vi "Car Simulation.vi"() -> ()   [LabVIEW 2020]
uses:
  <vilib>/event_ctls.llb/eventvkey.ctl
  <vilib>/numeric/Random Number (Range) I64.vi
  <vilib>/numeric/sub_Random U32.vi
panel:
  out "realdir":dbl format="%#_3g"
  in  "no road/road?":bool=TRUE
  out "velocity":cluster{"x":dbl, "y":dbl}
  in  "VKey 2":T1=enum."Ctrl"
  in  "Backward?":bool
  out "String":string
  out "location":T2
  out "readings":T3
  out "buffer":T4
  in  "y buffer":dbl
  in  "x buffer":dbl
  in  "end game":bool
  in  "Brake Pin":i32=2
  in  "Accelerator Pin":i32=1
  in  "xAccelerometer Pin":i32
  in  "Road Width":i8=7 min=5 max=11 step=2
  in  "Pause/Start":bool
  out "map":bool[][](array[boolean])
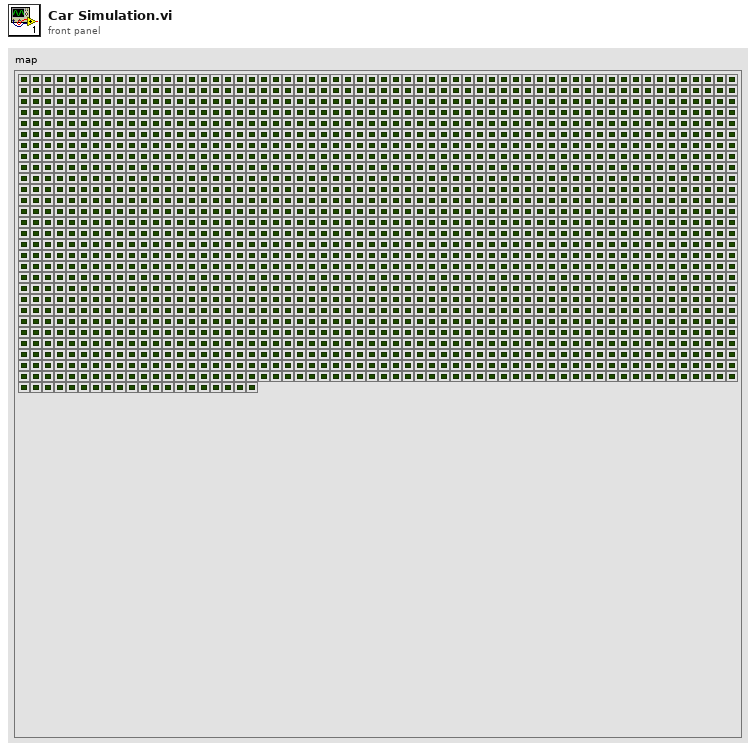
[diagram p1: front panel]
types:
  T1 = typedef "eventvkey.ctl" = enum16{"ASCII", "Enter", "Return", "Shift", "Ctrl", "Alt", "Cmd", "Opt", "Caps", "NumLock", "Clear", "Break", "Up", "Down", "Left", "Right", "Insert", "Delete", "Home", "End", "PageUp", "PageDown", "Escape", "Help", "Pause", "ScrollLock", "F1", "F2", "F3", "F4", "F5", "F6", "F7", "F8", "F9", "F10", "F11", "F12", "F13", "F14", "F15", "F16", "F17", "F18", "F19", "F20", "F21", "F22", "F23", "F24", "Play", "VolumeUp", "VolumeDown", "Mute", "Two Byte Char"}
  T2 = cluster{"Row":i64, "Column":i64, "Direction":i64}
  T3 = cluster{"xAccelerometer":dbl, "accelerator":dbl, "brake":dbl}
  T4 = cluster{"x buffer":dbl, "y buffer":dbl, "real direction":dbl}
  T5 = cluster{"number":i64, "number":i64, "number":i64}
  T6 = cluster{"Handle":i32, "xAccelerometer Pin":i32, "Accelerator Pin":i32, "Brake Pin":i32}
  T7 = cluster{"Row":i32, "Column":i32, "Direction":i32}
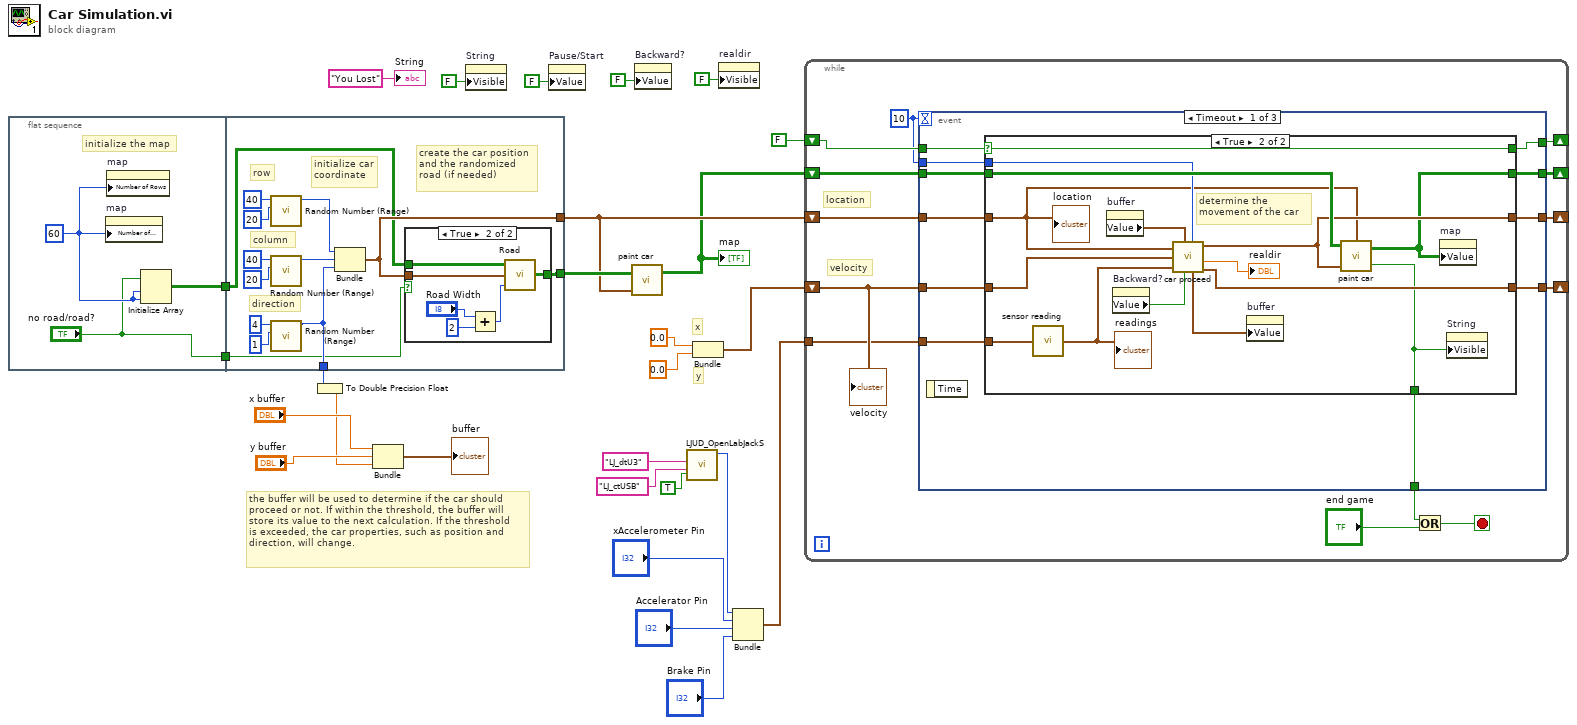
[diagram p0: block diagram]
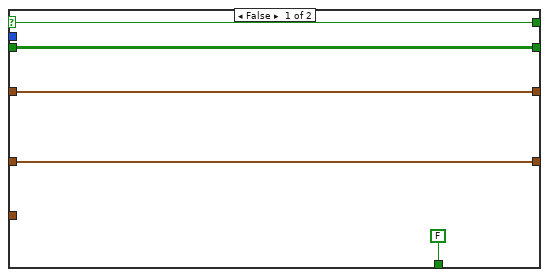
[diagram p2: hidden frame]
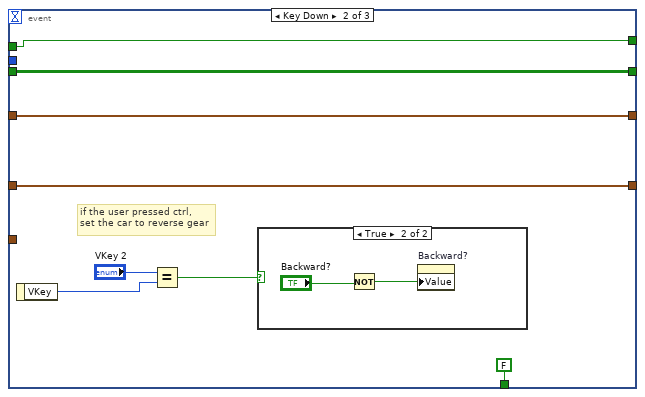
[diagram p3: hidden frame]
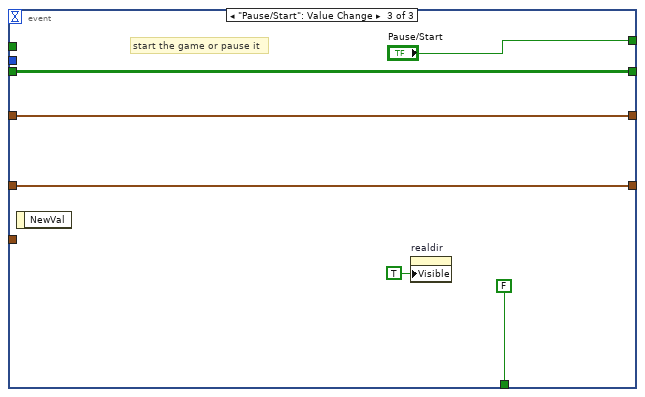
[diagram p5: hidden frame]
diagram:
  # "the buffer will be used to determine if the car should\nproceed or not. If within the threshold, the buffer will\nstore its value to the next calculation. If the threshold\nis exceeded, the car properties, such as position and\ndirection, will change."
  # "y"
  # "x"
  n1 = flat-sequence {
    tunnel: [w30] -> w26
    tunnel: ["no road/road?"] -> w9
    tunnel: [w36] -> w24
    tunnel: w26 -> [w35]
    tunnel: [w39] -> w25
    tunnel: [w34] -> w11
    tunnel: w9 -> [w31]
    frame #0 {
      w29 = u32 60 ("Number of Columns")
      # "initialize the map"
      n2 = property on="map" class="Arr (strict)"("Number of Columns"=w29) -> ()  [unwired: 2 in, 2 out]
      n3 = property on="map" class="Arr (strict)"("Number of Rows"=w29) -> ()  [unwired: 2 in, 2 out]
      n4 = Initialize Array("no road/road?", w29, w29) -> (w30:bool[][])
    }
    frame #1 {
      # "initialize car\ncoordinate"
      # "create the car position\nand the randomized\nroad (if needed)"
      # "direction"
      # "column"
      # "row"
      n5 = call-poly <vilib>:"Random Number (Range).vi"("lower bound (-100)"=i64 20, "upper bound (100)"=i64 40) -> ("number"=w38:i64)  [unwired: 9 in]
      n6 = call-poly <vilib>:"Random Number (Range).vi"("lower bound (-100)"=i64 20, "upper bound (100)"=i64 40) -> ("number"=w37:i64)  [unwired: 9 in]
      n7 = call-poly <vilib>:"Random Number (Range).vi"("lower bound (-100)"=i64 1, "upper bound (100)"=i64 4) -> ("number"=w34:i64)  [unwired: 9 in]
      n8 = Bundle("number"=w38, "number"=w37, "number"=w34) -> (w36:T5)  [unwired: 1 in]
      n9 = case shown="True" w31 {
        tunnel: [w44 w50] -> w39
        tunnel: w36 -> [_ w46]
        tunnel: w35 -> [w44 w45]
        frame False {
        }
        frame True {
          n10 = Add(x="Road Width", y=i8 2) -> (x+y=w47:i8)
          n11 = call "Road.vi"("Road Width"=w47, "coordinate"=w46, "Map in"=w45) -> ("Map out"=w50:bool[][])
        }
      }
    }
  }
  n12 = To Double Precision Float(number=w11) -> (double precision float=w10:dbl)
  n13 = Bundle("x buffer"="x buffer", "y buffer"="y buffer", w10) -> (→"buffer":cluster{"x buffer":dbl, "y buffer":dbl, dbl})  [unwired: 1 in]
  n14 = property on="String" class="Str"("Visible"=FALSE) -> ()  [unwired: 2 in, 2 out]
  n15 = property on="Pause/Start" class="Bool (strict)"("Value"=FALSE ("Start/Stop")) -> ()  [unwired: 2 in, 2 out]
  n16 = call "paint car.vi"("New Location"=w24, "Map in"=w25) -> ("Map out"=w15:bool[][])  [unwired: 2 in, 1 out]
  "map" <- w15
  n17 = property on="Backward?" class="Bool (strict)"("Value"=FALSE ("Backward?")) -> ()  [unwired: 2 in, 2 out]
  n18 = call <vilib>:"LJUD_OpenLabJackS.vi"("FirstFound"=TRUE, "ConnectionType"="LJ_ctUSB", "DeviceType"="LJ_dtU3") -> ("Handle"=w2:i32)  [unwired: 6 in, 2 out]
  n19 = Bundle("element"=0.0, "element"=0.0) -> (w20:cluster{"element":dbl, "element":dbl})  [unwired: 1 in]
  n20 = property on="realdir" class="DigNum (strict)"("Visible"=FALSE) -> ()  [unwired: 2 in, 2 out]
  n21 = Bundle("Handle"=w2, "xAccelerometer Pin"="xAccelerometer Pin", "Accelerator Pin"="Accelerator Pin", "Brake Pin"="Brake Pin") -> (w23:T6)  [unwired: 1 in]
  n22 = while {
    shift-right: [w63] -> _
    shift-left: FALSE ("Start/Stop") -> [w62]
    shift-right: [w58] -> _
    shift-left: w24 -> [w61]
    shift-right: [w57] -> _
    shift-left: w20 -> [w60]
    tunnel: w23 -> [w59]
    shift-right: [w54] -> _
    shift-left: w15 -> [w55]
    stop <- w52 stop-if-true
    w56 = 10
    # "velocity"
    # "location"
    n23 = event shown="[0] Timeout" {
      selector: _ -> [_ _ _]
      dyn-events: _ -> [_ _ _]
      timeout: w56 -> [_ _ _]
      tunnel: [w73 w102 "Pause/Start"] -> w63
      tunnel: w62 -> [w74 w102 _]
      tunnel: w61 -> [w72 w100 w108]
      tunnel: w60 -> [w71 w99 w107]
      tunnel: w59 -> [w70 _ _]
      tunnel: [w69 w100 w108] -> w58
      tunnel: [w68 w99 w107] -> w57
      tunnel: w56 -> [w67 _ _]
      tunnel: w55 -> [w66 w101 w109]
      tunnel: [w65 w101 w109] -> w54
      tunnel: [w64 FALSE ("hit?") FALSE ("hit?")] -> w51
      event Timeout {
        n24 = event-data() -> ()  [unwired: 1 in, 1 out]
        n25 = case shown="True" w74 {
          selector: w74 -> [w79 w94]
          tunnel: [w79 w94] -> w73
          tunnel: w72 -> [w78 w83]
          tunnel: w71 -> [w77 w92]
          tunnel: w70 -> [_ w93]
          tunnel: [w78 w87] -> w69
          tunnel: [w77 w89] -> w68
          tunnel: w67 -> [_ w84]
          tunnel: w66 -> [w76 w88]
          tunnel: [w76 w86] -> w65
          tunnel: [FALSE ("hit?") w85] -> w64
          frame False {
          }
          frame True {
            # "determine the\nmovement of the car"
            n26 = call "sensor reading.vi"("Input parameter"=w93) -> ("readings"=w91:T3)
            "readings" <- w91
            n27 = property on="buffer" class="Clust (strict)"() -> ("Value"=w90:T4)  [unwired: 2 in, 2 out]
            n28 = property on="Backward?" class="Bool (strict)"() -> ("Value"=w81:bool)  [unwired: 2 in, 2 out]
            n29 = call "car proceed.vi"("location in"=w83, "old buffer"=w90, "velocity in"=w92, "sensor reading"=w91, "Backward?"=w81, "refresh rate"=w84) -> ("location out"=w87:T7, "new buffer"=w82:T4, "realdir"=→"realdir":dbl, "velocity out"=w89:cluster{"x":dbl, "y":dbl})  [unwired: 1 in]
            n30 = property on="buffer" class="Clust (strict)"("Value"=w82) -> ()  [unwired: 2 in, 2 out]
            n31 = call "paint car.vi"("Old Location"=w83, "New Location"=w87, "Map in"=w88) -> ("hit?"=w85:bool, "Map out"=w86:bool[][])  [unwired: 1 in]
            n32 = property on="map" class="Arr (strict)"("Value"=w86) -> ()  [unwired: 2 in, 2 out]
            n33 = property on="String" class="Str"("Visible"=w85) -> ()  [unwired: 2 in, 2 out]
            "location" <- w83
          }
        }
      }
      event Key Down {
        # "if the user pressed ctrl,\nset the car to reverse gear"
        n34 = event-data() -> ("VKey"=w96:T1)  [unwired: 1 in]
        n35 = Equal?(x="VKey 2", y=w96) -> (x = y?=w95:bool)
        n36 = case shown="True" w95 {
          frame False {
          }
          frame True {
            n37 = Not(x="Backward?") -> (.not. x?=w103:bool)
            n38 = property on="Backward?" class="Bool (strict)"("Value"=w103) -> ()  [unwired: 2 in, 2 out]
          }
        }
      }
      event "Pause/Start": Value Change {
        # "start the game or pause it"
        n39 = event-data() -> ()  [unwired: 1 in, 1 out]
        n40 = property on="realdir" class="DigNum (strict)"("Visible"=TRUE) -> ()  [unwired: 2 in, 2 out]
      }
    }
    n41 = Or(x=w51, y="end game") -> (x .or. y?=w52:bool)
    "velocity" <- w60
  }
  "String" <- "You Lost" ("String")
